vi "build.flowToVarient.io-write.vi"(8 "error in":errorcluster, 9 "flow params":string[](array[string]), 11 "Step in":variant) -> (0 "error out":errorcluster, 3 "variant out":variant)   [LabVIEW 2024]
uses:
  controls/type.StepFunction.ctl
  controls/typeStepVarients.ctl
  Polymorphics/variantCtrlStepFunction.vi
  Polymorphics/variantCtrlString.vi
  proc.util.validateParamExist.vi
  <vilib>/Utility/error.llb/Clear Errors.vi
  util.error.create.vi
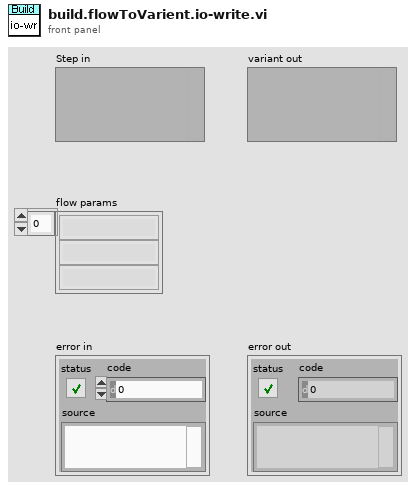
[diagram p1: front panel]
types:
  T1 = typedef "typeStepVarients.ctl" = enum16{"stepNameID", "stepFunction", "stepReport", "stepSetpoint", "stepPointer", "stepProcPointer", "stepIoPointer", "stepIoValue", "stepFilePointer", "stepMessage", "stepTimeString", "stepNumReg", "stepStrReg", "stepSeconds", "stepUnitDoseParams", "stepUnitIndex"}
  T2 = typedef "type.StepFunction.ctl" = enum16{"__NO-OP", "_DELAY_LOAD", "_DELAY_COMPARE", "_JUMP", "_COMPLETE", "_COMPARE", "_LOG_MESSAGE", "_LOG_LAST_REPORT", "_SCHEDULE", "_SCHED_DAILY", "CLK_COMPARE", "PROC_START", "PROC_STOP", "PROC_LOAD", "PROC_COMPLETION_CHECK", "PROC_COMPLETION_LOAD", "_IO_READ", "_IO_READ_MANY", "_IO_WRITE", "_IO_WRITE_BY_REG", "_IO_GET_OUTPUT", "_OCS_CHECK", "_OCS_RECORD", "_GET_RH", "_GET_ACC_UV", "_GET_WD", "_GET_WS", "_REC_DELETE", "_REC_MOVE", "_REC_COPY", "_IRR_CHECK", "UNIT_CHECK", "UNIT_SAMPLE", "UNIT_DOSE"}
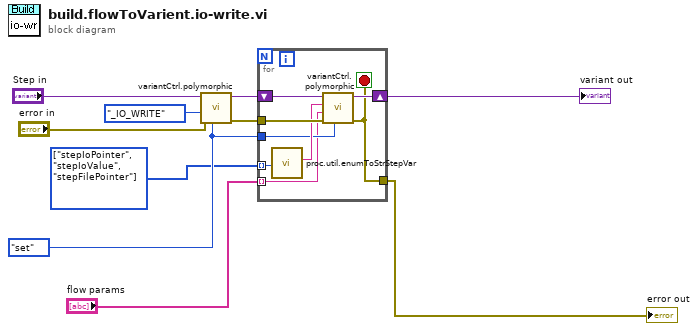
[diagram p0: block diagram]
diagram:
  w7 = enum16{"get", "set"}."set" ("get/set")
  w5 = T1[] [enum."stepIoPointer", enum."stepIoValue", enum."stepFilePointer"] items=["stepNameID", "stepFunction", "stepReport", "stepSetpoint", "stepPointer", "stepProcPointer", "stepIoPointer", "stepIoValue", "stepFilePointer", "stepMessage", "stepTimeString", "stepNumReg", "stepStrReg", "stepSeconds", "stepUnitDoseParams", "stepUnitIndex"] ("Step var")
  n1 = call-poly "variantCtrl.polymorphic.vi"("menu in (get)"=w7, "error in"="error in", "StepFunction"=type.StepFunction."_IO_WRITE" ("Operation out"), "variant in"="Step in") -> ("error out"=w2:errorcluster, "variant out"=w3:variant)  [unwired: 4 in, 2 out]
  n2 = for {
    tunnel: w5 -> [w16] mode=indexing
    tunnel: w7 -> [w14]
    tunnel: "flow params" -> [w13] mode=indexing
    shift-right: [w12] -> w9
    shift-left: w3 -> [w17]
    tunnel: w2 -> [w18]
    tunnel: [w11] -> w6
    stop <- w11 stop-if-true
    n3 = call "proc.util.enumToStrStepVar.vi"("Step var"=w16) -> ("String"=w15:string)  [unwired: 10 in]
    n4 = call-poly "variantCtrl.polymorphic.vi"("menu in (get)"=w14, "error in"=w18, "String Value"=w13, "name in"=w15, "Step in"=w17) -> ("error out"=w11:errorcluster, "Step out"=w12:variant)  [unwired: 3 in, 2 out]
  }
  "variant out" <- w9
  "error out" <- w6
